vi "Get Measurements.vi"(0 "reference in":refnum<class "Simulated-PowerModule.lvclass">, 11 "Error In":errorcluster) -> (4 "reference out":refnum<class "Simulated-PowerModule.lvclass">, 6 "measurements":T1[](array[typedef]), 15 "Error Out":errorcluster)   [LabVIEW 2023, in "Simulated-PowerModule.lvlib" / "Simulated-PowerModule.lvclass"]
uses:
  Simulated-PowerModule.lvclass
  builds/PowerModuleInterface/home/lvuser/natinst/bin/PowerModuleInterface.lvlibp/Classes/PowerModule_interface/Measurements.ctl
  builds/PowerModuleInterface/home/lvuser/natinst/bin/PowerModuleInterface.lvlibp/Classes/PowerModule_interface/PowerModuleInterface.lvclass
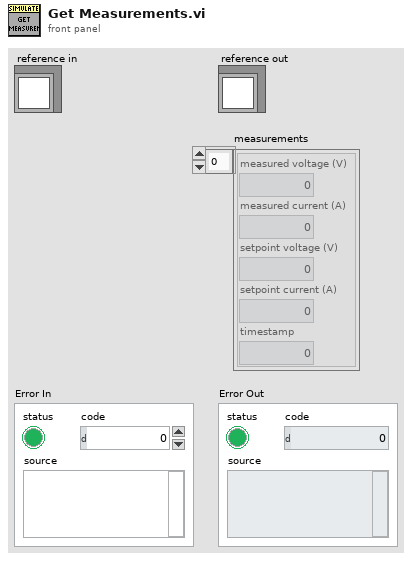
[diagram p1: front panel]
types:
  T1 = typedef "PowerModuleInterface.lvlibp/PowerModuleInterface.lvclass/Measurements.ctl" = cluster{"measured voltage (V)":dbl, "measured current (A)":dbl, "setpoint voltage (V)":dbl, "setpoint current (A)":dbl, "timestamp":dbl}
  T2 = typedef "Simulated-PowerModule.lvlib/Simulated-PowerModule.lvclass/ObjectAttributes.ctl" = cluster{"JSON Config Path":path, "Configuration":T3, "connected":bool, "reserved":bool, "energized":bool, "output enabled":bool, "Mode":T4, "Range":T5, "Slew Rates":T6, "Setpoints":cluster{"voltage":dbl, "current":dbl, "resistance":dbl}, "Measurements":cluster{"voltage":dbl, "current":dbl, "resistance":dbl}, "Limits":T7, "active faults":string[], "fault":bool, "profile":dbl[][], "step dt":i64}
  T3 = typedef "Simulated-PowerModule.lvlib/Simulated-PowerModule.lvclass/Configuration.ctl" = cluster{"IP Address":string}
  T4 = typedef "Simulated-PowerModule.lvlib/Simulated-PowerModule.lvclass/Mode.ctl" = u16
  T5 = typedef "PowerModuleInterface.lvlibp/PowerModuleInterface.lvclass/Range.ctl" = cluster{"Current Max (A)":dbl, "Current Min (A)":dbl, "Voltage Max (V)":dbl, "Voltage Min (V)":dbl}
  T6 = typedef "PowerModuleInterface.lvlibp/PowerModuleInterface.lvclass/Slew Rates.ctl" = cluster{"Current Decrease (A/sec)":dbl, "Current Increase (A/sec)":dbl, "Voltage Decrease (V/sec)":dbl, "Voltage Increase (V/sec)":dbl, "Resistance Decrease (Ohm/sec)":dbl, "Resistance Increase (Ohm/sec)":dbl}
  T7 = typedef "PowerModuleInterface.lvlibp/PowerModuleInterface.lvclass/Limits.ctl" = cluster{"Current Max (A)":dbl, "Current Min (A)":dbl, "Voltage Max (V)":dbl, "Voltage Min (V)":dbl, "Power Max (W)":dbl, "Power Min (W)":dbl}
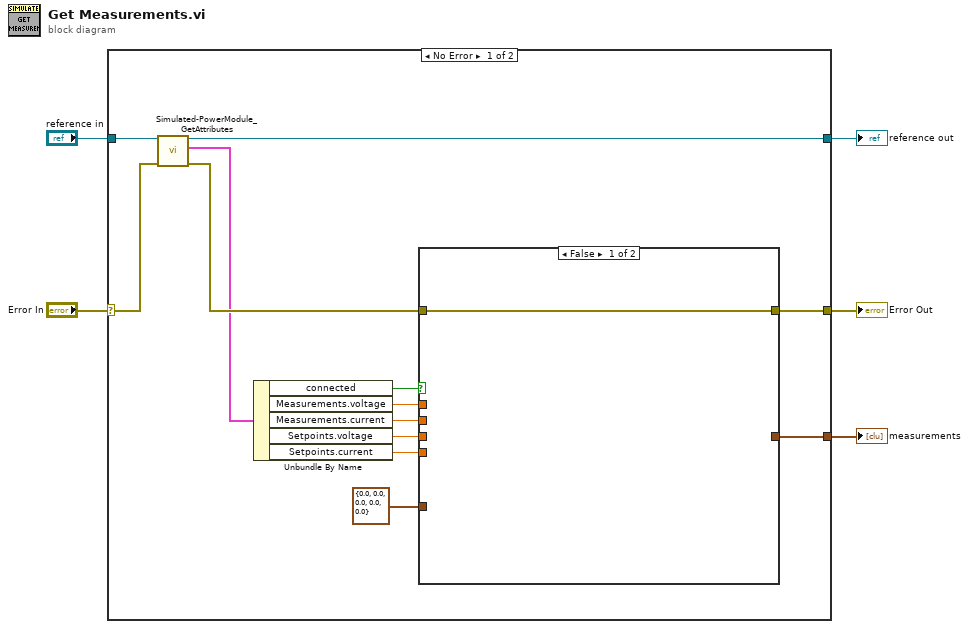
[diagram p0: block diagram]
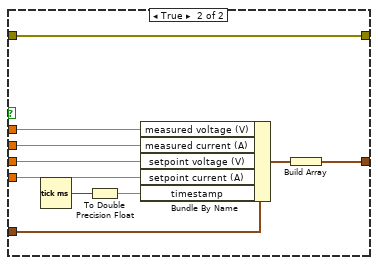
[diagram p2: hidden frame]
diagram:
  n1 = case shown="No Error" "Error In" {
    selector: "Error In" -> [w17 w30]
    tunnel: "reference in" -> [w18 w31]
    tunnel: [w14 w31] -> w5
    tunnel: [w15 w30] -> w2
    tunnel: [w13 _] -> w1
    frame No Error {
      n2 = call "Simulated-PowerModule_GetAttributes.vi"("reference in"=w18, "Error In"=w17) -> ("reference out"=w14:refnum<class "Simulated-PowerModule.lvclass">, "Data"=w10:T2, "Error Out"=w16:errorcluster)  [unwired: 10 in, 1 out]
      n3 = Unbundle By Name(w10) -> ("connected"=w12:bool, "Measurements.voltage"=w9:dbl, "Measurements.current"=w8:dbl, "Setpoints.voltage"=w7:dbl, "Setpoints.current"=w6:dbl)
      n4 = case shown="False" w12 {
        tunnel: w16 -> [w19 w29]
        tunnel: [w19 w29] -> w15
        tunnel: T1 {"measured voltage (V)"=0.0, "measured current (A)"=0.0, "setpoint voltage (V)"=0.0, "setpoint current (A)"=0.0, "timestamp"=0.0} ("Measurements") -> [_ w28]
        tunnel: [_ w27] -> w13
        tunnel: w9 -> [_ w23]
        tunnel: w8 -> [_ w22]
        tunnel: w7 -> [_ w21]
        tunnel: w6 -> [_ w20]
        frame False {
        }
        frame True {
          n5 = Tick Count (ms)() -> (millisecond timer value=w24:u32)
          n6 = To Double Precision Float(number=w24) -> (double precision float=w26:dbl)
          n7 = Bundle By Name(cluster=w28, "measured voltage (V)"=w23, "measured current (A)"=w22, "setpoint voltage (V)"=w21, "setpoint current (A)"=w20, "timestamp"=w26) -> (w25:T1)
          n8 = Build Array(w25) -> (w27:T1[])
        }
      }
    }
    frame Error {
    }
  }
  "Error Out" <- w2
  "reference out" <- w5
  "measurements" <- w1
